vi "Set Main Data.vi"(8 "error in (no error)":errorcluster caption="entrée d'erreur (pas d'erreur)", 10 "Main_Data Read":T1(array[cluster]), 11 "Database Altyor en entrée":refnum<class "Database Altyor.lvclass">) -> (0 "error out":errorcluster caption="sortie d'erreur", 3 "Database Altyor en sortie":refnum<class "Database Altyor.lvclass">)   [LabVIEW 2020, in "Library Instrument & Equipement.lvlib" / "Library Database.lvlib" / "Database Altyor.lvclass"]
uses:
  Database Altyor.lvclass
  Database Altyor.lvclass/Database Altyor.ctl
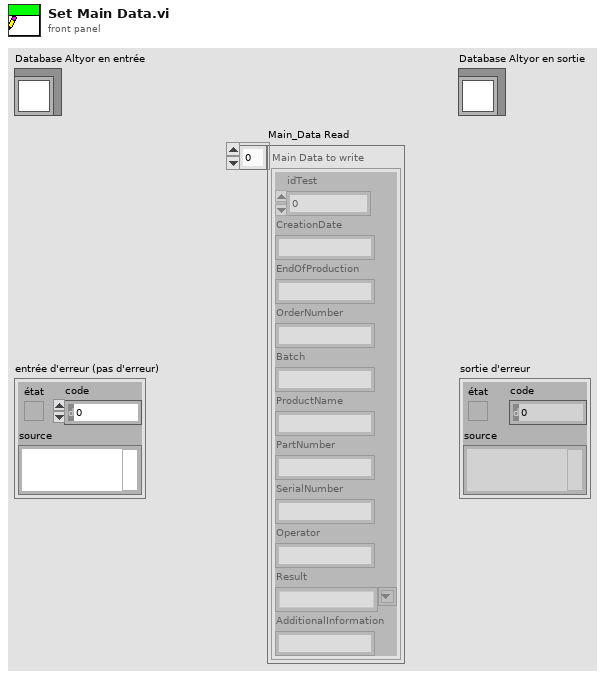
[diagram p1: front panel]
types:
  T1 = cluster{"idTest":u32, "CreationDate":string, "EndOfProduction":string, "OrderNumber":string, "Batch":string, "ProductName":string, "PartNumber":string, "SerialNumber":string, "Operator":string, "Result":string, "AdditionalInformation":string}[]
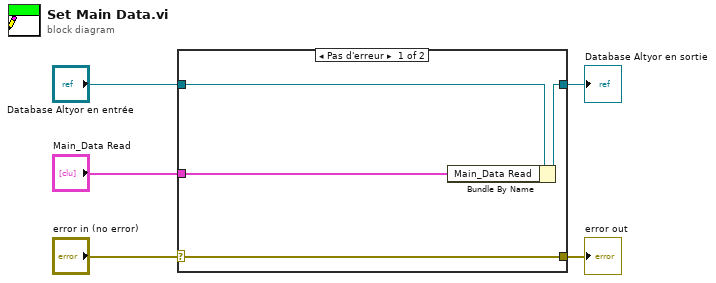
[diagram p0: block diagram]
diagram:
  n1 = case shown="Pas d'erreur" "error in (no error)" {
    selector: "error in (no error)" -> [w9 w10]
    tunnel: [w9 w10] -> w4
    tunnel: [w7 w11] -> w2
    tunnel: "Database Altyor en entrée" -> [w8 w11]
    tunnel: "Main_Data Read" -> [w6 _]
    frame No Error {
      n2 = Bundle By Name(cluster=w8, "Main_Data Read"=w6) -> (w7:refnum<class "Database Altyor.lvclass">)
    }
    frame Error {
    }
  }
  "error out" <- w4
  "Database Altyor en sortie" <- w2
